vi "Read Difftrack.lvclass.vi"(8 "error in (no error)":errorcluster, 11 "TargetDef.lvclass in":refnum<class "TargetDef.lvclass">) -> (0 "error out":errorcluster, 2 "Difftrack.lvclass":refnum<class "Difftrack.lvclass">, 3 "TargetDef.lvclass out":refnum<class "TargetDef.lvclass">)   [LabVIEW 2009]
uses:
  TargetDef/TargetDef.lvclass
  Difftrack.lvclass
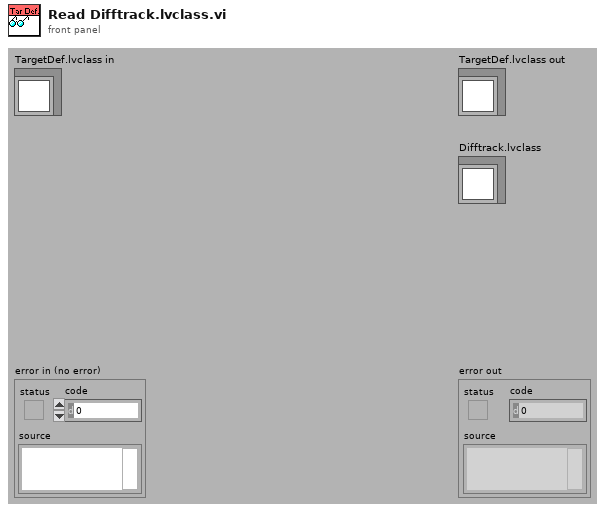
[diagram p1: front panel]
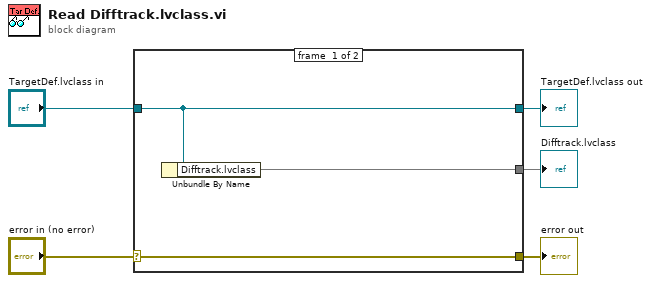
[diagram p0: block diagram]
diagram:
  n1 = case shown="No Error" "error in (no error)" {
    selector: "error in (no error)" -> [w8 w9]
    tunnel: [w8 w9] -> w4
    tunnel: [w7 w10] -> w2
    tunnel: "TargetDef.lvclass in" -> [w7 w10]
    tunnel: [w6 _] -> w1
    frame #0 {
      n2 = Unbundle By Name(w7) -> ("Difftrack.lvclass"=w6)
    }
    frame #1 {
    }
  }
  "error out" <- w4
  "TargetDef.lvclass out" <- w2
  "Difftrack.lvclass" <- w1
